vi "cRIO Test ftp webDAV installed.vi"(6 "Connect Timeout (4000 ms)":u32=4000 caption="Verbindungs-Timeout (4000 ms)", 7 "PC":bool, 8 "error in (no error)":errorcluster, 9 "Password":string="iag", 10 "User Name":string="iag", 11 "System Session Ref":refnum<k21>="cRIO-9068 (10.1.128.164)") -> (0 "error out":errorcluster, 1 "WebDAV":bool, 3 "ftp":bool, 4 "Runtimes":string[](array[string]))   [LabVIEW 2020, in "FTP WebDAV.lvlib"]
uses:
  FTP WebDAV.lvlib
  <vilib>/nisyscfg/Get Installed Components.vi
  <vilib>/nisyscfg/Close (System).vi
  <vilib>/nisyscfg/nisyscfg.lvlib
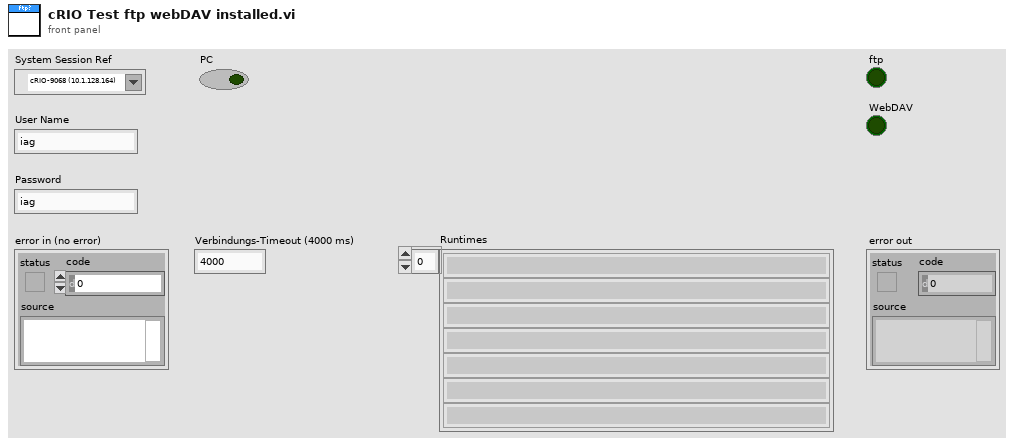
[diagram p1: front panel]
types:
  T1 = typedef "nisyscfg.lvlib/Software 1.2.ctl" = cluster{"title":string, "description":string, "ID":string, "version":string, "component type":T2}
  T2 = typedef "nisyscfg.lvlib/Component Type.ctl" = u32
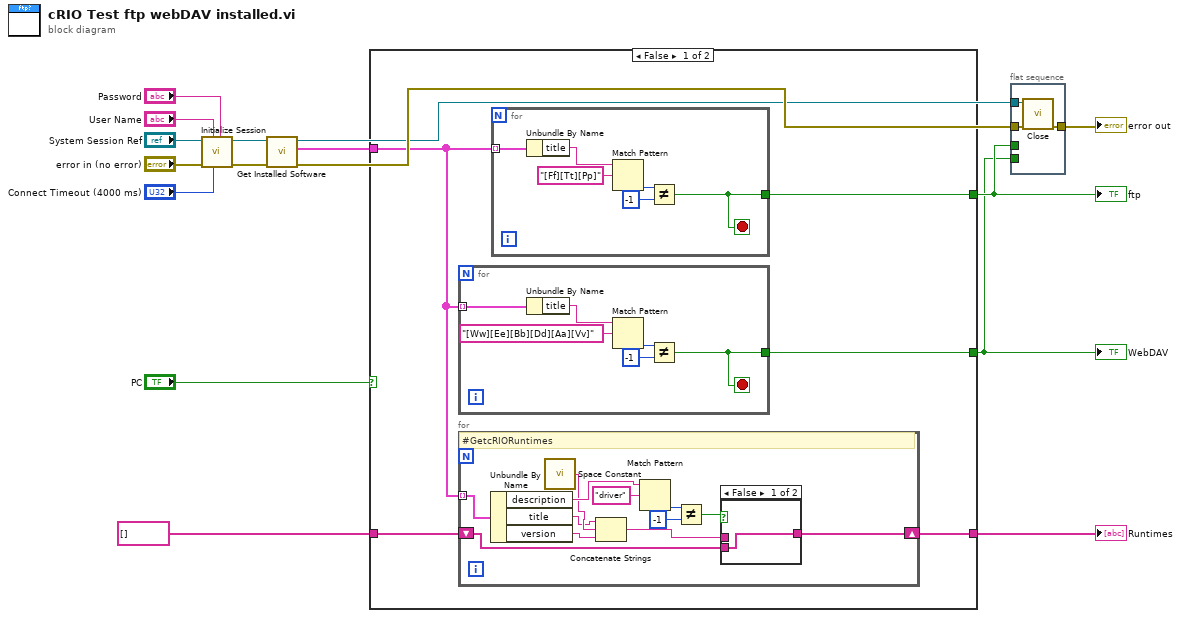
[diagram p0: block diagram]
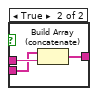
[diagram p2: hidden frame]
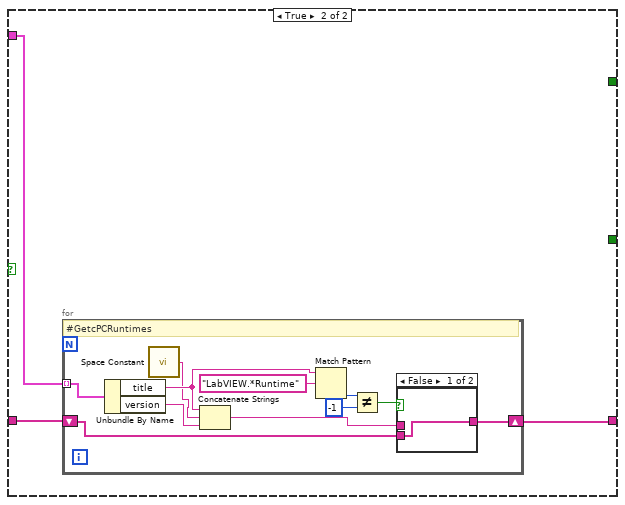
[diagram p3: hidden frame]
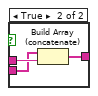
[diagram p4: hidden frame]
diagram:
  n1 = call <vilib>:"Initialize Session.vi"("Password"="Password", "Connect Timeout (4000 ms)"="Connect Timeout (4000 ms)", "User Name"="User Name", "error in (no error)"="error in (no error)", "Target (localhost)"="System Session Ref") -> ("error out"=w15:errorcluster, "Session out"=w16:refnum<k21>)  [unwired: 5 in]
  n2 = call-poly <vilib>:"Get Installed Software.vi"("error in (no error)"=w15, "Session in"=w16) -> ("error out"=w14:errorcluster, "Software Components"=w4:T1[], "Session out"=w13:refnum<k21>)  [unwired: 7 in]
  n3 = case shown="False" "PC" {
    tunnel: [w21 _] -> w12
    tunnel: [w20 _] -> w11
    tunnel: w4 -> [w19 w50]
    tunnel: [w18 w51] -> w3
    tunnel: string[] [] -> [w17 w52]
    frame False {
      n4 = for {
        tunnel: w19 -> [w43] mode=indexing
        tunnel: [w38] -> w20
        stop <- w38 stop-if-true
        n5 = Unbundle By Name(w43) -> ("title"=w42:string)
        n6 = Match Pattern(string=w42, regular expression="[Ww][Ee][Bb][Dd][Aa][Vv]" ("Regulärer Ausdruck")) -> (offset past match=w40:i32)  [unwired: 1 in, 3 out]
        n7 = Not Equal?(x=w40, y=-1) -> (x != y?=w38:bool)
      }
      n8 = for {
        tunnel: w19 -> [w30] mode=indexing
        shift-right: [w27] -> w18
        shift-left: w17 -> [w26]
        # "#GetcRIORuntimes"
        n9 = Unbundle By Name(w30) -> ("description"=w28:string, "title"=w22:string, "version"=w23:string)
        n10 = call <vilib>:"Space Constant.vi"() -> ("String"=w24:string)
        n11 = Concatenate Strings(w22, w24, w23) -> (w25:string)
        n12 = Match Pattern(string=w28, regular expression="driver" ("Regulärer Ausdruck")) -> (offset past match=w32:i32)  [unwired: 1 in, 3 out]
        n13 = Not Equal?(x=w32, y=-1) -> (x != y?=w29:bool)
        n14 = case shown="False" w29 {
          tunnel: w25 -> [_ w37]
          tunnel: [w34 w36] -> w27
          tunnel: w26 -> [w34 w35]
          frame False {
          }
          frame True {
            n15 = Build Array (concatenate)(w35, w37) -> (w36:string[])
          }
        }
      }
      n16 = for {
        tunnel: w19 -> [w49] mode=indexing
        tunnel: [w44] -> w21
        stop <- w44 stop-if-true
        n17 = Unbundle By Name(w49) -> ("title"=w48:string)
        n18 = Match Pattern(string=w48, regular expression="[Ff][Tt][Pp]" ("Regulärer Ausdruck")) -> (offset past match=w46:i32)  [unwired: 1 in, 3 out]
        n19 = Not Equal?(x=w46, y=-1) -> (x != y?=w44:bool)
      }
    }
    frame True {
      n20 = for {
        tunnel: w50 -> [w60] mode=indexing
        shift-right: [w57] -> w51
        shift-left: w52 -> [w56]
        # "#GetcPCRuntimes"
        n21 = Unbundle By Name(w60) -> ("title"=w58:string, "version"=w54:string)
        n22 = call <vilib>:"Space Constant.vi"() -> ("String"=w53:string)
        n23 = Concatenate Strings(w58, w53, w54) -> (w55:string)
        n24 = Match Pattern(string=w58, regular expression="LabVIEW.*Runtime" ("Regulärer Ausdruck")) -> (offset past match=w62:i32)  [unwired: 1 in, 3 out]
        n25 = Not Equal?(x=w62, y=-1) -> (x != y?=w59:bool)
        n26 = case shown="False" w59 {
          tunnel: w55 -> [_ w67]
          tunnel: [w64 w66] -> w57
          tunnel: w56 -> [w64 w65]
          frame False {
          }
          frame True {
            n27 = Build Array (concatenate)(w65, w67) -> (w66:string[])
          }
        }
      }
    }
  }
  "ftp" <- w12
  "WebDAV" <- w11
  "Runtimes" <- w3
  n28 = flat-sequence {
    tunnel: w14 -> [w70]
    tunnel: w13 -> [w69]
    tunnel: w12 -> [_]
    tunnel: w11 -> [_]
    tunnel: [w68] -> w6
    frame #0 {
      n29 = call-poly <vilib>:"Close.vi"("error in (no error)"=w70, "Session in"=w69) -> ("error out"=w68:errorcluster)  [unwired: 9 in]
    }
  }
  "error out" <- w6
